vi "Update Chassis Firmware.vi"(0 "session in":refnum<k21>, 1 "username":string, 2 "password":string, 5 "chassis":refnum<k21>, 7 "firmware path":path, 11 "error in (no error)":errorcluster, 12 "connect timeout (10 sec)":dbl=10.0) -> (4 "session out":refnum<k21>, 15 "error out":errorcluster)   [LabVIEW 2020, in "SLSC.lvlib"]
doc: "Updates the firmware of the chassis."
uses:
  <vilib>/SLSC/SLSC.lvlib
  <vilib>/nisyscfg/Upgrade Firmware (File).vi
  <vilib>/nisyscfg/Close (Resources).vi
  <vilib>/nisyscfg/Close (Filter).vi
  <vilib>/nisyscfg/nisyscfg.lvlib
  <resource>/objmgr/nisysapi.rc
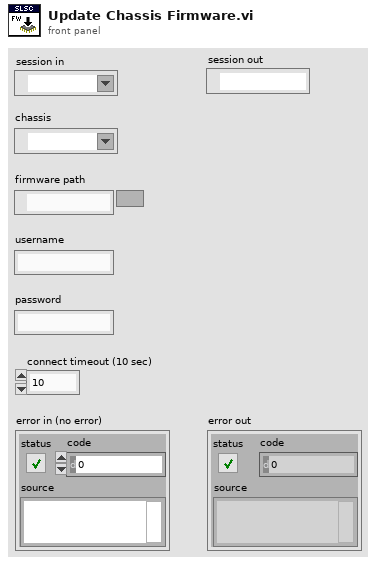
[diagram p1: front panel]
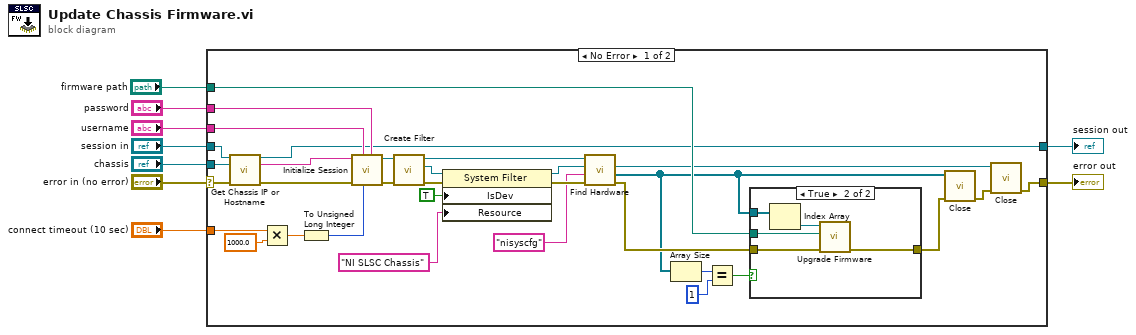
[diagram p0: block diagram]
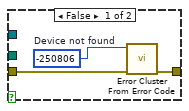
[diagram p2: hidden frame]
diagram:
  n1 = case shown="No Error" "error in (no error)" {
    selector: "error in (no error)" -> [w10 w51]
    tunnel: "chassis" -> [w15 _]
    tunnel: "username" -> [w31 _]
    tunnel: "password" -> [w30 _]
    tunnel: "connect timeout (10 sec)" -> [w29 _]
    tunnel: "firmware path" -> [w19 _]
    tunnel: [w16 w51] -> w3
    tunnel: "session in" -> [w14 w50]
    tunnel: [w13 w50] -> w1
    frame No Error {
      n2 = call <vilib>:"Get Chassis IP or Hostname.vi"("session in"=w14, "chassis"=w15, "error in (no error)"=w10) -> ("session out"=w13:refnum<k21>, "chassis IP address/hostname"=w12:string, "error out"=w11:errorcluster)  [unwired: 10 in]
      n3 = Multiply(x=w29, y=1000.0) -> (x*y=w26:dbl)
      n4 = To Unsigned Long Integer(number=w26) -> (unsigned 32bit integer=w27:u32)
      n5 = call <vilib>:"Initialize Session.vi"("Password"=w30, "Connect Timeout (4000 ms)"=w27, "User Name"=w31, "error in (no error)"=w11, "Target (localhost)"=w12) -> ("error out"=w37:errorcluster, "Session out"=w35:refnum<k21>)  [unwired: 5 in]
      n6 = call <vilib>:"Create Filter.vi"("error in (no error)"=w37, "Session in"=w35) -> ("error out"=w33:errorcluster, "Filter out"=w34:refnum<k20>, "Session out"=w36:refnum<k21>)  [unwired: 7 in]
      n7 = property class="System Filter"(reference=w34, error in=w33, "IsDev"=TRUE ("Is Device"), "Resource"="NI SLSC Chassis" ("y")) -> (reference out=w39:refnum<k20>, error out=w38:errorcluster)
      n8 = call <vilib>:"Find Hardware.vi"("error in (no error)"=w38, "Experts"="nisyscfg", "Filter in"=w39, "Session in"=w36) -> ("error out"=w20:errorcluster, "Resources out"=w18:refnum<k20>[], "Filter out"=w17:refnum<k20>)  [unwired: 4 in, 1 out]
      n9 = Array Size(array=w18) -> (size(s)=w25:i32)
      n10 = Equal?(x=w25, y=1) -> (x = y?=w23:bool)
      n11 = case shown="True" w23 {
        tunnel: [w42 w49] -> w22
        tunnel: w20 -> [w43 w45]
        tunnel: w18 -> [_ w48]
        tunnel: w19 -> [_ w47]
        frame False {
          w44 = -250806  # Device not found
          n12 = call <vilib>:"Error Cluster From Error Code.vi"("error in (no error)"=w43, "error code (0)"=w44) -> ("error out"=w42:errorcluster)  [unwired: 7 in]
        }
        frame True {
          n13 = Index Array(array=w48) -> (element=w46:refnum<k20>)  [unwired: 1 in]
          n14 = call-poly <vilib>:"Upgrade Firmware.vi"("error in (no error)"=w45, "Firmware File"=w47, "Resource in"=w46) -> ("error out"=w49:errorcluster)  [unwired: 5 in, 3 out]
        }
      }
      n15 = call-poly <vilib>:"Close.vi"("error in (no error)"=w22, "Resources in"=w18) -> ("error out"=w21:errorcluster)  [unwired: 9 in]
      n16 = call-poly <vilib>:"Close.vi"("error in (no error)"=w21, "Filter in"=w17) -> ("error out"=w16:errorcluster)  [unwired: 9 in]
    }
    frame Error {
    }
  }
  "error out" <- w3
  "session out" <- w1
